vi "MALT Output Get One.vi"(8 "error in":errorcluster, 9 "Port":i32, 10 "Address":i32, 11 "MALT FamilyCode":T1=enum."MALT132") -> (0 "error out":errorcluster, 3 "Status":bool)   [LabVIEW 2018, in "AltonTech MALT200817.lvlib"]
uses:
  <instrlib>/AltonTech MALT/AltonTech MALT200817.lvlib
  <instrlib>/AltonTech MALT/Public/Types/MALT CardTypes.ctl
panel:
  out "Response":string
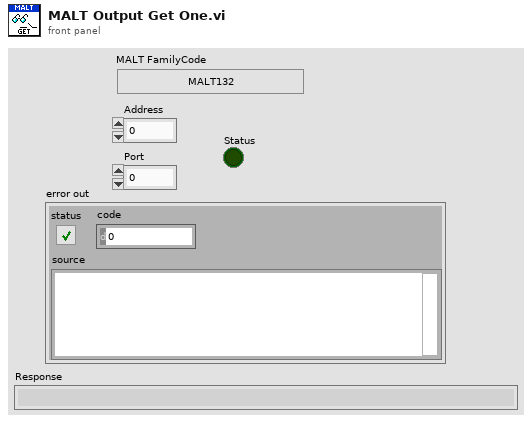
[diagram p1: front panel]
types:
  T1 = typedef "AltonTech MALT200817.lvlib/MALT CardTypes.ctl" = enum32{"-", "YAV90832", "YAV904X8", "MALT132", "YAV91616", "YAV90PIN", "YAV90096", "YAV90HVT", "YAV90CLR", "YAV90128", "YAV90PNE", "YAVCANCON", "YAV91775", "YAV90XXX", "YAV90MMU", "H730050", "H710060", "H710061", "YAV90304", "MMI", "YAV90060", "MALT160T", "YAV90059", "Not Defined"}
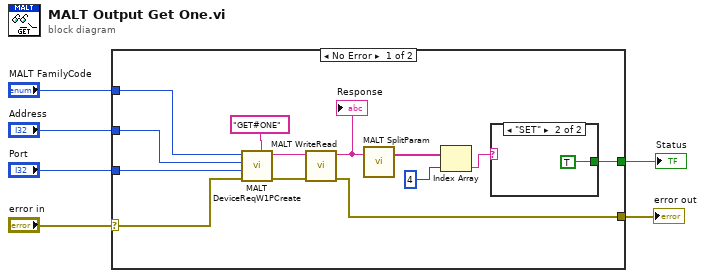
[diagram p0: block diagram]
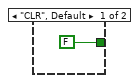
[diagram p2: hidden frame]
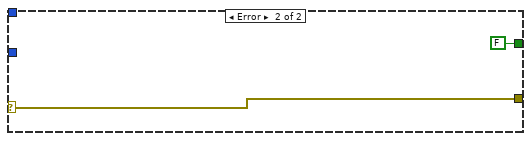
[diagram p3: hidden frame]
diagram:
  n1 = case shown="No Error" "error in" {
    selector: "error in" -> [w8 w23]
    tunnel: [w18 w23] -> w6
    tunnel: [w14 FALSE] -> w5
    tunnel: "Address" -> [w12 _]
    tunnel: "MALT FamilyCode" -> [w9 _]
    tunnel: "Port" -> [w7 _]
    frame No Error {
      n2 = call <instrlib>:"MALT DeviceReqW1PCreate.vi"("Cmd"="GET#ONE" ("cmd"), "error in"=w8, "Param1"=w7, "Address"=w12, "FamilyCode"=w9) -> ("error out"=w11:errorcluster, "Request"=w13:string)  [unwired: 4 in]
      n3 = call <instrlib>:"MALT WriteRead.vi"("error in"=w11, "Request"=w13) -> ("error out"=w18:errorcluster, "Response"=w19:string)  [unwired: 8 in]
      "Response" <- w19
      n4 = call <instrlib>:"MALT SplitParam.vi"("Line"=w19) -> ("Items"=w17:string[])  [unwired: 2 in]
      n5 = Index Array(array=w17, index=4) -> (element=w15:string)
      n6 = case shown="\"SET\"" w15 {
        tunnel: [FALSE TRUE] -> w14
        frame "CLR", Default {
        }
        frame "SET" {
        }
      }
    }
    frame Error {
    }
  }
  "error out" <- w6
  "Status" <- w5
